vi "Render Inverted Section.vi"(8 "Error In":errorcluster) -> (0 "Error Out":errorcluster)   [LabVIEW 2018, in "Tests.lvlib" / "Render.lvlib"]
uses:
  Render.lvlib
  src/Toolkit/Data/Array/Array.lvclass
  D:/Users/cfield/Code/Field R&D Services/Mustache/trunk/src/Toolkit/Data/Abstract/Abstract.lvclass
  src/Toolkit/Data/Map/Map.lvclass
  src/Toolkit/Low-Level/Support/Lex String.vi
  src/Toolkit/Data/Map/Support/From Datum.vi
  src/Toolkit/Low-Level/Support/Render to String.vi
  <vilib>/addons/_JKI Toolkits/Caraya/classes/Test/Test.lvclass
  <vilib>/addons/_JKI Toolkits/Caraya/classes/Assert/Assert.lvclass
  src/Toolkit/Toolkit.lvlib
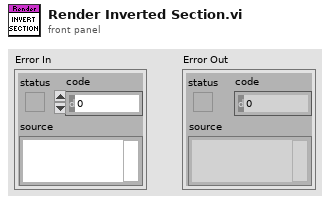
[diagram p1: front panel]
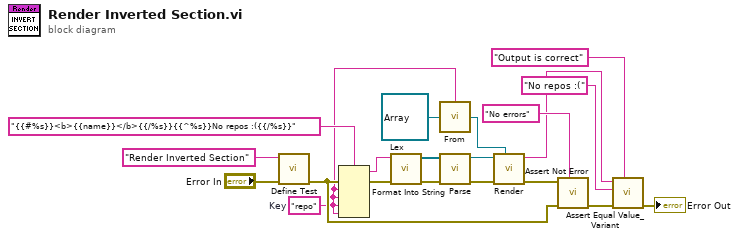
[diagram p0: block diagram]
diagram:
  w3 = "repo"  # Key
  n1 = call <vilib>:"Define Test.vi"("error in (no error)"="Error In", "Label (VI Title)"="Render Inverted Section") -> ("error out"=w8:errorcluster)  [unwired: 9 in]
  n2 = Format Into String(format string="{{#%s}}<b>{{name}}</b>{{/%s}}{{^%s}}No repos :({{/%s}}", error in=w8, w3, w3, w3, w3) -> (resulting string=w5:string, error out=w7:errorcluster)  [unwired: 1 in]
  n3 = call-poly "Lex.vi"("Error In"=w7, "Input"=w5) -> ("Error Out"=w10:errorcluster, "Tokens"=w11:refnum<class "Abstract.lvclass">[])  [unwired: 8 in]
  n4 = call-poly "From.vi"("Value"=refnum<class "Array.lvclass"> refnum ("Toolkit.lvlib:Data.lvlib:Array.lvclass"), "Key"=w3) -> ("Map"=w9:refnum<class "Map.lvclass">)
  n5 = call "Parse.vi"("Error In"=w10, "Tokens"=w11) -> ("Error Out"=w12:errorcluster, "Abstract Syntax Tree"=w1:refnum<class "Root.lvclass">)  [unwired: 8 in]
  n6 = call-poly "Render.vi"("Data"=w9, "Error In"=w12, "Abstract Syntax Tree"=w1) -> ("Error Out"=w14:errorcluster, "Output"=w13:string)  [unwired: 7 in]
  n7 = call <vilib>:"Assert Not Error.vi"("Label"="No errors", "error in (no error)"=w8, "Not Error?"=w14) -> ("error out"=w17:errorcluster)  [unwired: 8 in]
  n8 = call <vilib>:"Assert Equal Value_Variant.vi"("Label"="Output is correct", "error in (no error)"=w17, "Y"="No repos :(", "X"=w13) -> ("error out"=→"Error Out":errorcluster)  [unwired: 7 in]
